vi "GetControlRef[Poly].vi"   [LabVIEW 2016, in "Drona.lvlib" / "GetControlRef.lvlib"]
doc: "Gives the reference of the control which is specified"
uses:
  GetControlRef/GetControlRef.lvlib
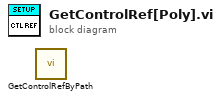
[diagram p0: block diagram]
diagram:
  n1 = call "GetControlRefByPath.vi"() -> ()  [unwired: 13 in, 3 out]
